vi "CleanUp.vi"(0 "object in":refnum<class "AD2_SDK.lvclass">, 5 "error in (no error)":errorcluster) -> (14 "object out":refnum<class "AD2_SDK.lvclass">, 19 "error out":errorcluster)   [LabVIEW 2023, in "AD2_SDK.lvclass"]
uses:
  AD2_SDK.lvclass
  AD2_SDK.lvclass/AD2_SDK.ctl
  Olasdwf/Olasdwf.lvlib
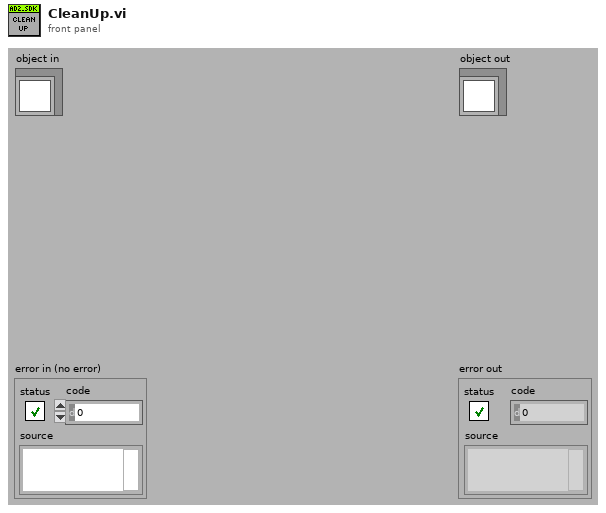
[diagram p1: front panel]
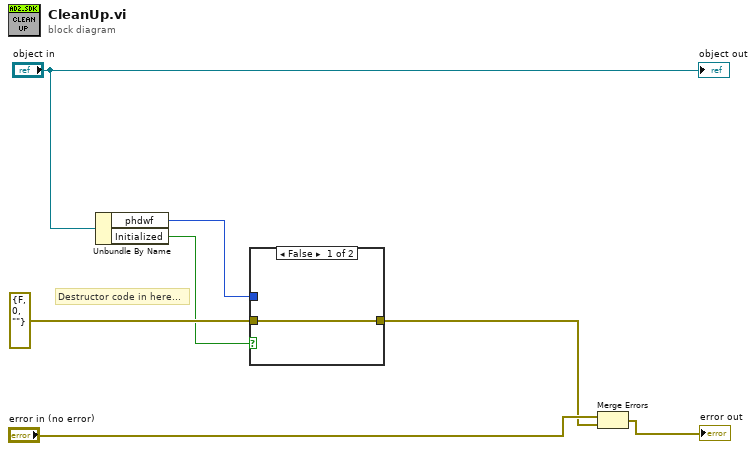
[diagram p0: block diagram]
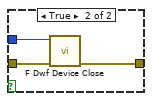
[diagram p2: hidden frame]
diagram:
  # "Destructor code in here..."
  n1 = Unbundle By Name("object in") -> ("phdwf"=w6:i32, "Initialized"=w1:bool)
  n2 = case shown="False" w1 {
    tunnel: w6 -> [_ w11]
    tunnel: errorcluster {"status"=FALSE, "code"=0, "source"=""} ("error in (no error)") -> [w8 w10]
    tunnel: [w8 w9] -> w4
    frame False {
    }
    frame True {
      n3 = call "F Dwf Device Close.vi"("error in (no error)"=w10, "hdwf"=w11) -> ("error out"=w9:errorcluster)  [unwired: 8 in, 1 out]
    }
  }
  n4 = Merge Errors("error in (no error)", w4) -> (→"error out":errorcluster)
  "object out" <- "object in"
